vi "Unreserve Trig0 Line.vi"(6 "Backplane refs":refnum<visa-resource-name>[](array[refnum]), 8 "error in (no error)":errorcluster) -> (0 "error out":errorcluster)   [LabVIEW 2011, in "PXIe-433x Custom Device.lvlib"]
uses:
  PXIe-433x Custom Device.lvlib
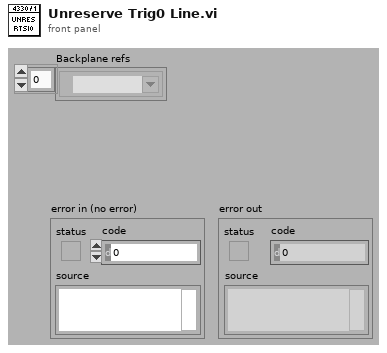
[diagram p1: front panel]
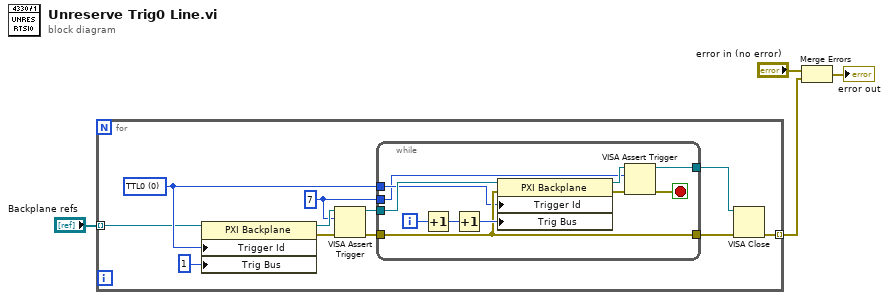
[diagram p0: block diagram]
diagram:
  n1 = for {
    tunnel: "Backplane refs" -> [w9] mode=indexing
    tunnel: [w5] -> w2 mode=indexing
    w8 = u16 7 ("protocol (default:  0)")
    w10 = i16 0 items=["Software"=-1, "TTL0"=0, "TTL1"=1, "TTL2"=2, "TTL3"=3, "TTL4"=4, "TTL5"=5, "TTL6"=6, "TTL7"=7, "ECL0"=8, "ECL1"=9] ("General Settings:Trigger Identifier")
    n2 = property class="PXI Backplane"(reference=w9, "Trigger Id"=w10, "Trig Bus"=i16 1 ("PXI/PCI Settings:Trigger Bus Number")) -> (reference out=w13:refnum<visa-resource-name>, error out=w14:errorcluster)  [unwired: 1 in]
    n3 = VISA Assert Trigger(8:w14, 10:w8, 11:w13) -> (0:w11:errorcluster, 3:w12:refnum<visa-resource-name>)
    n4 = while {
      tunnel: [w23] -> w7
      tunnel: w12 -> [w26]
      tunnel: w11 -> [w23]
      tunnel: [w19] -> w6
      tunnel: w10 -> [w18]
      tunnel: w8 -> [w17]
      i -> [w25]
      stop <- w20 stop-if-true
      n5 = Increment(x=w25) -> (x+1=w16:i32)
      n6 = Increment(x=w16) -> (x+1=w24:i32)
      n7 = property class="PXI Backplane"(reference=w26, error in=w23, "Trigger Id"=w18, "Trig Bus"=w24) -> (reference out=w21:refnum<visa-resource-name>, error out=w22:errorcluster)
      n8 = VISA Assert Trigger(8:w22, 10:w17, 11:w21) -> (0:w20:errorcluster, 3:w19:refnum<visa-resource-name>)
    }
    n9 = VISA Close(VISA resource name=w6, error in (no error)=w7) -> (error out=w5:errorcluster)
  }
  n10 = Merge Errors("error in (no error)", w2) -> (→"error out":errorcluster)
